vi "WFPropertiesAssemble.vi"(8 "Duration (s)":dbl, 9 "Ramp (s)":dbl, 10 "Amplitude (V)":dbl, 11 "Fs (Hz)":dbl min=0.0) -> (3 "Waveform Properties":T1 {"Ramp (s)" min=0.0; "Fs (Hz)" min=0.0})   [LabVIEW 2009]
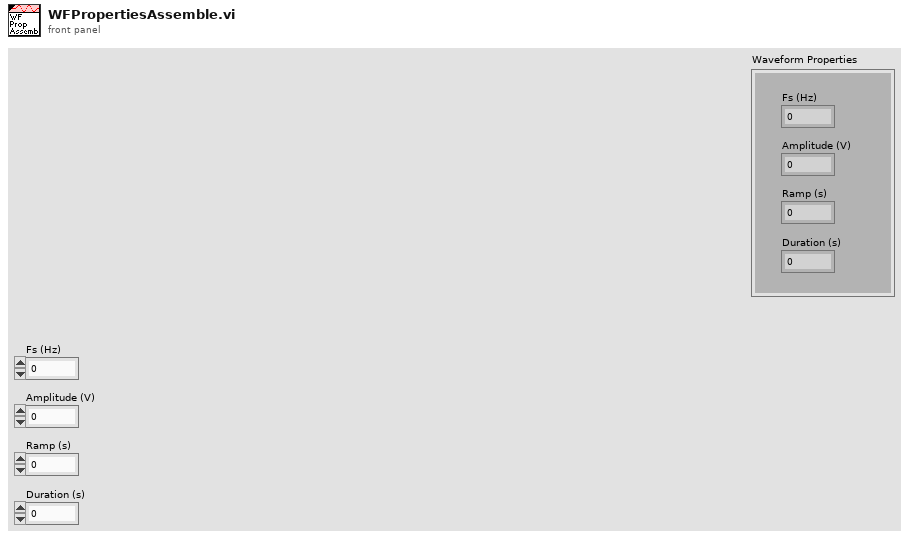
[diagram p1: front panel]
types:
  T1 = cluster{"Fs (Hz)":dbl, "Amplitude (V)":dbl, "Ramp (s)":dbl, "Duration (s)":dbl}
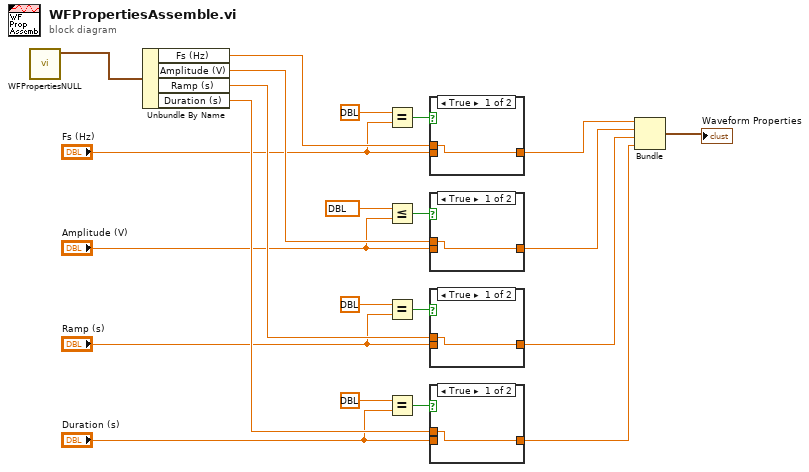
[diagram p0: block diagram]
diagram:
  n1 = call "WFPropertiesNULL.vi"() -> ("Waveform Properties"=w1:T1)  [unwired: 11 in]
  n2 = Unbundle By Name(w1) -> ("Fs (Hz)"=w8:dbl, "Amplitude (V)"=w12:dbl, "Ramp (s)"=w15:dbl, "Duration (s)"=w20:dbl)
  n3 = Equal?(x=dbl ?, y="Fs (Hz)") -> (x = y?=w10:bool)
  n4 = Less Or Equal?(x=dbl ?, y="Amplitude (V)") -> (x <= y?=w14:bool)
  n5 = Equal?(x=dbl ?, y="Ramp (s)") -> (x = y?=w18:bool)
  n6 = Equal?(x=dbl ?, y="Duration (s)") -> (x = y?=w22:bool)
  n7 = case shown="True" w10 {
    tunnel: "Fs (Hz)" -> [_ w24]
    tunnel: [w23 w24] -> w7
    tunnel: w8 -> [w23 _]
    frame #0 {
    }
    frame #1 {
    }
  }
  n8 = case shown="True" w14 {
    tunnel: "Amplitude (V)" -> [_ w26]
    tunnel: [w25 w26] -> w11
    tunnel: w12 -> [w25 _]
    frame #0 {
    }
    frame #1 {
    }
  }
  n9 = case shown="True" w18 {
    tunnel: "Ramp (s)" -> [_ w28]
    tunnel: [w27 w28] -> w16
    tunnel: w15 -> [w27 _]
    frame #0 {
    }
    frame #1 {
    }
  }
  n10 = case shown="True" w22 {
    tunnel: "Duration (s)" -> [_ w30]
    tunnel: w20 -> [w29 _]
    tunnel: [w29 w30] -> w19
    frame #0 {
    }
    frame #1 {
    }
  }
  n11 = Bundle("Fs (Hz)"=w7, "Amplitude (V)"=w11, "Ramp (s)"=w16, "Duration (s)"=w19) -> (→"Waveform Properties":T1)  [unwired: 1 in]
